vi "ConvertVariousStrToVariousStr.vi"(9 "out various type":enum16{"hex", "asc"}(ring), 10 "input various type":enum16{"hex", "asc"}(ring), 11 "various str in":string) -> (3 "various str out":string)   [LabVIEW 2018, in "Library-DataConvert.lvlib"]
uses:
  Library-DataConvert.lvlib
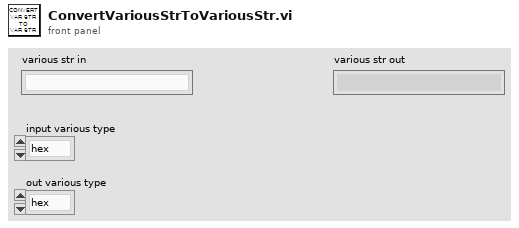
[diagram p1: front panel]
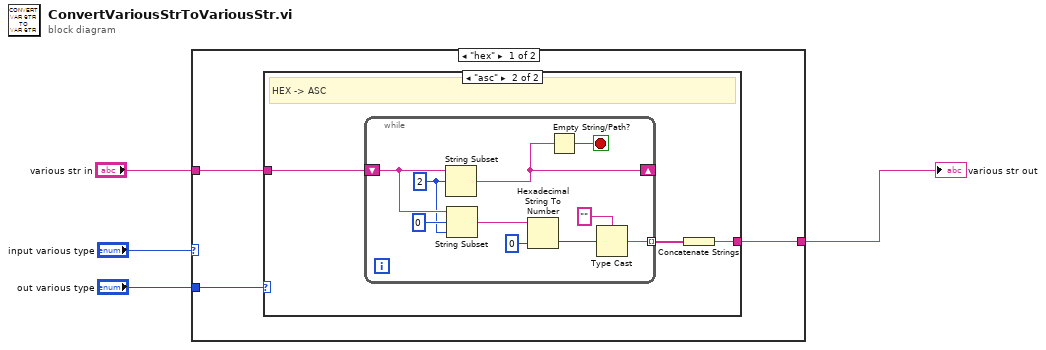
[diagram p0: block diagram]
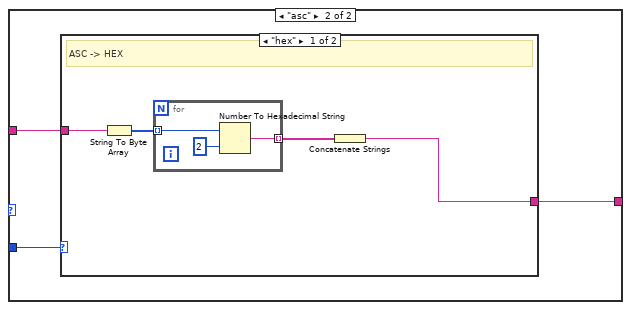
[diagram p3: hidden frame]
diagram:
  n1 = case shown="\"hex\"" "input various type" {
    tunnel: "various str in" -> [w7 w24]
    tunnel: [w6 w23] -> w2
    tunnel: "out various type" -> [w5 w22]
    frame "hex" {
      n2 = case shown="\"asc\"" w5 {
        tunnel: w7 -> [w8 w11]
        tunnel: [w8 w9] -> w6
        frame "hex", Default {
          # "HEX -> HEX (BY PASS)"
        }
        frame "asc" {
          # "HEX -> ASC"
          n3 = while {
            shift-right: [w20] -> _
            shift-left: w11 -> [w21]
            tunnel: [w12] -> w10 mode=indexing
            stop <- w19 stop-if-true
            w17 = 2 ("오프셋(0)")
            n4 = String Subset(string=w21, offset (0)=w17) -> (substring=w20:string)  [unwired: 1 in]
            n5 = String Subset(string=w21, offset (0)=0 ("오프셋(0)"), length (rest)=w17) -> (substring=w16:string)
            n6 = Hexadecimal String To Number(string=w16, default (0uL)=u8 0 ("기본(0 U32)")) -> (number=w13:u8)  [unwired: 1 in, 1 out]
            n7 = Empty String/Path?(string/path=w20) -> (empty?=w19:bool)
            n8 = Type Cast(type="", x=w13) -> (*(type *) &x=w12:string)
          }
          n9 = Concatenate Strings(w10) -> (w9:string)
        }
      }
    }
    frame "asc" {
      n10 = case shown="\"hex\"" w22 {
        tunnel: w24 -> [w28 w32]
        tunnel: [w25 w32] -> w23
        frame "hex" {
          # "ASC -> HEX"
          n11 = String To Byte Array(string=w28) -> (unsigned byte array=w27:u8[])
          n12 = for {
            tunnel: w27 -> [w31] mode=indexing
            tunnel: [w30] -> w26 mode=indexing
            n13 = Number To Hexadecimal String(1:i16 2 ("폭(-)"), 2:w31) -> (0:w30:string)
          }
          n14 = Concatenate Strings(w26) -> (w25:string)
        }
        frame "asc", Default {
          # "ASC -> ASC (BY PASS)"
        }
      }
    }
  }
  "various str out" <- w2
